vi "pl1000SetTrigger.vi"(0 "pl1000 handle":i16, 1 "Trigger":T1={"Enabled"=FALSE, "AutoTrigger"=FALSE, "delay (%)"=-50.0, "Auto Trigger\nTiime (ms)"=1000, "Channel"=1, "Trigger Direction"=0, "threshold (mV)"=500, "hysteresis (mV)"=5} {"Trigger Direction" items=["rising edge", "falling edge"]; "Channel" items=["Ch1"=1, "Ch2"=2, "Ch3"=3, "Ch4"=4, "Ch5"=5, "Ch6"=6, "Ch7"=7, "Ch8"=8, "Ch9"=9, "Ch10"=10, "Ch11"=11, "Ch12"=12, "Ch13"=13, "Ch14"=14, "Ch15"=15, "Ch16"=16]}, 3 "maxValue":u16, 11 "error in (no error)":errorcluster) -> (4 "pl1000 handle out":i16, 15 "error out":errorcluster)   [LabVIEW 2010]
doc: "This function sets up the trigger, which controls when the unit starts capturing data\n\nenabled: whether to enable or disable the trigger:\n\nauto_trigger: whether or not to re-arm the trigger automatically after each trigger event:\n\nauto_ms: time in milliseconds after which the unit will auto-trigger if the trigger condition is not met\n\nchannel: which channel to trigger on\n\ndir: which edge to trigger on\n\nthreshold: trigger threshold (the level at which the trigger will activate) in ADC counts\n\nhysteresis: trigger hysteresis in ADC counts. This is the difference between the upper and lower thresholds. The signal must then pass through both thresholds in the same direction in order to activate the trigger, so that there are fewer unwanted trigger events caused by noise. The minimum value allowed is 1. \n\ndelay: delay between the trigger event and the start of the block as a percentage of the block size. 0% means that the trigger event is the first data value in the block, and -50% means that the trigger event is in the middle of the block."
uses:
  pl1000.dll
panel:
  # "Trigger delay of \n-50% means the\ntrigger event is\nin the middle of \nthe block"
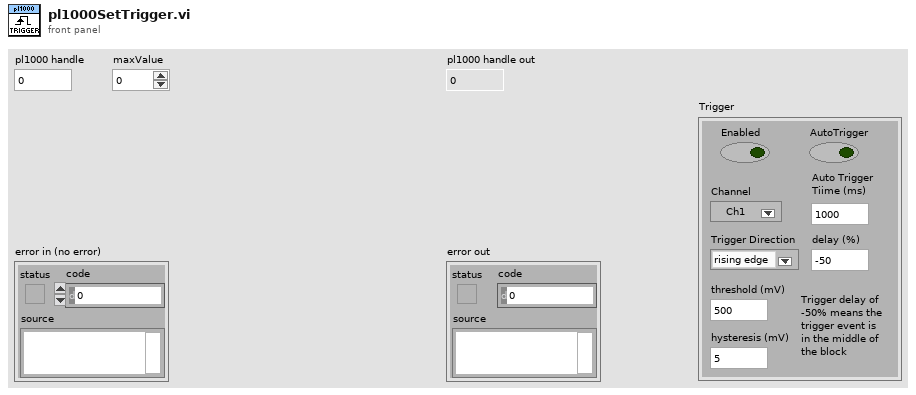
[diagram p1: front panel]
types:
  T1 = cluster{"Enabled":bool, "AutoTrigger":bool, "delay (%)":sgl, "Auto Trigger\nTiime (ms)":u16, "Channel":u16, "Trigger Direction":u16, "threshold (mV)":u16, "hysteresis (mV)":u16}
  T2 = cluster{"status":bool, "code":u32, "source":string}
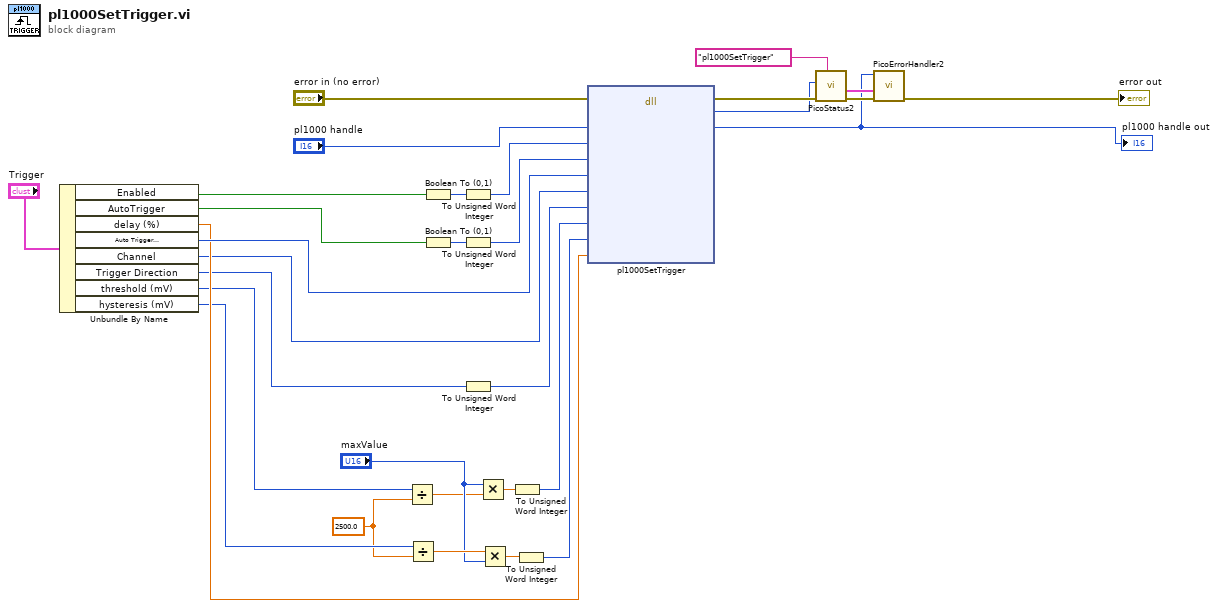
[diagram p0: block diagram]
diagram:
  w2 = 2500.0 ("y")
  n1 = Unbundle By Name("Trigger") -> ("Enabled"=w14:bool, "AutoTrigger"=w13:bool, "delay (%)"=w11:sgl, "Auto Trigger\nTiime (ms)"=w12:u16, "Channel"=w10:u16, "Trigger Direction"=w9:u16, "threshold (mV)"=w3:u16, "hysteresis (mV)"=w8:u16)
  n2 = Divide(x=w3, y=w2) -> (x/y=w1:dbl)
  n3 = Divide(x=w8, y=w2) -> (x/y=w6:dbl)
  n4 = Boolean To (0,1)(Boolean=w14) -> (0, 1=w29:i16)
  n5 = Boolean To (0,1)(Boolean=w13) -> (0, 1=w27:i16)
  n6 = To Unsigned Word Integer(number=w29) -> (unsigned 16bit integer=w28:u16)
  n7 = To Unsigned Word Integer(number=w27) -> (unsigned 16bit integer=w26:u16)
  n8 = To Unsigned Word Integer(number=w9) -> (unsigned 16bit integer=w25:u16)
  n9 = Multiply(x="maxValue", y=w1) -> (x*y=w4:dbl)
  n10 = Multiply(x=w6, y="maxValue") -> (x*y=w7:dbl)
  n11 = To Unsigned Word Integer(number=w4) -> (unsigned 16bit integer=w17:u16)
  n12 = To Unsigned Word Integer(number=w7) -> (unsigned 16bit integer=w16:u16)
  n13 = dll-call lib="pl1000.dll" fn="pl1000SetTrigger"(error in="error in (no error)", "handle"="pl1000 handle", "enabled"=w28, "autoTrigger"=w26, "autoMs"=w12, "channel"=w10, "dir"=w25, "threshold"=w17, "hysteresis"=w16, "delay"=w11) -> (error out=w21:errorcluster, "status"=w19:u32, "handle"=w18:i16)  [unwired: 10 in, 1 out]
  "pl1000 handle out" <- w18
  n14 = call "PicoStatus2.vi"("PICO source"="pl1000SetTrigger", "Error in"=w21, "PICO STATUS"=w19) -> ("error out"=w24:errorcluster, "PICO_STATUS out"=w23:T2)  [unwired: 5 in]
  n15 = call "PicoErrorHandler2.vi"("error in (no error)"=w24, "PICO_STATUS in"=w23, "handle In"=w18) -> ("error out"=→"error out":errorcluster)  [unwired: 8 in]
